vi "Analyze.vi"(8 "error in (no error)":errorcluster, 10 "Image in":T1, 11 "Analyze FF Spectrum in":refnum<class "Analyze FF Spectrum.lvclass">) -> (0 "error out":errorcluster, 1 "Result":refnum<class "Analyze Results Base.lvclass">, 2 "Image out":T1, 3 "Analyze FF Spectrum out":refnum<class "Analyze FF Spectrum.lvclass">)   [LabVIEW 2020, in "Analyze.lvlib" / "Analyze FF Spectrum.lvclass"]
uses:
  Analyze FF Spectrum.lvclass
  C:/POLARIS Programme/POLARIS-AS-3-Cams/Submodules/HIJ Vision/Analyze/Analyze Classes/Analyze BaseClass/Analyze BaseClass/Analyze BaseClass.lvclass
  <vilib>/vision/Image Controls.llb/IMAQ Image.ctl
  Results and Overlays/Results Base/Analyze Results Base.lvclass
  Results and Overlays/Results SRFF/Analyze Results FF-Spectrum.lvclass
  C:/POLARIS Programme/POLARIS-AS-3-Cams/Submodules/HIJ Vision/Analyze/Results and Overlays/Results Base/Analyze Results Base.lvclass
  Analyze Parameter/Analyze Parameter Spectral Calibration/Analyze Parameter Spectral Calibration.lvclass
  C:/POLARIS Programme/POLARIS-AS-3-Cams/Submodules/HIJ Vision/Analyze/Analyze Parameter/Analyze Parameter Base/Analyze Parameter Base.lvclass
  Results and Overlays/Results SRFF/Analyze Results FF-Spectrum.lvclass/Analyze Results FF-Spectrum.ctl
  Results and Overlays/Results SRFF/Write SRFF Spectrum.vi
  Analyze BaseClass/Analyze BaseClass/Analyze BaseClass.lvclass
  <vilib>/vision/NI_Vision_Development_Module.lvlib
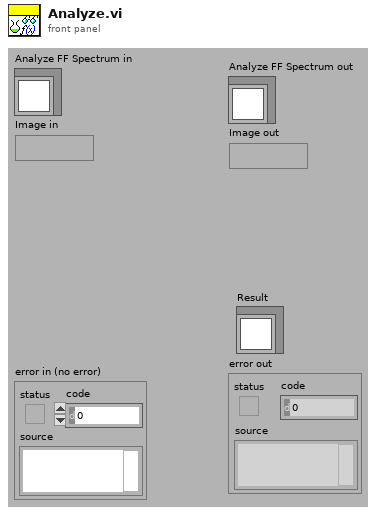
[diagram p1: front panel]
types:
  T1 = typedef "IMAQ Image.ctl" = refnum<image>
  T2 = typedef "Image Type" = u32
  T3 = typedef "ROI Descriptor" = cluster{"Global Rectangle":i32[], "Contours":cluster{"ID":enum32{"External", "Internal"}, "Type":u32, "Coordinates":i32[]}[]}
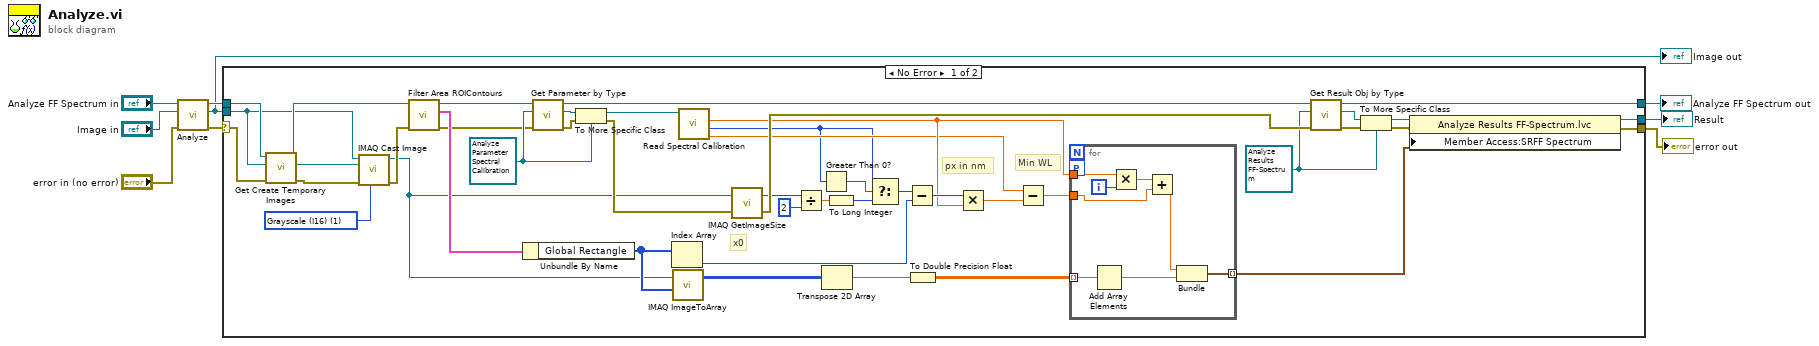
[diagram p0: block diagram]
diagram:
  n1 = call-parent "Analyze.vi"("error in (no error)"="error in (no error)", "Image in"="Image in", "Analyze BaseClass in"="Analyze FF Spectrum in") -> ("error out"=w1:errorcluster, "Image out"=w6:T1, "Analyze BaseClass out"=w7:refnum<class "Analyze FF Spectrum.lvclass">)  [unwired: 5 in, 1 out]
  "Image out" <- w6
  n2 = case shown="No Error" w1 {
    selector: w1 -> [w17 w64]
    tunnel: w7 -> [w18 w63]
    tunnel: w6 -> [w13 _]
    tunnel: [w34 _] -> w4
    tunnel: [w33 w64] -> w3
    tunnel: [w24 w63] -> w2
    frame No Error {
      w11 = T2 1 items=["Grayscale (U8)", "Grayscale (I16)", "Grayscale (SGL)", "Complex (CSG)", "RGB (U32)", "HSL (U32)", "RGB (U64)", "Grayscale (U16)"] ("Image Type")
      w29 = refnum<class "Analyze Parameter Spectral Calibration.lvclass"> refnum ("Spectral Calibration")
      w21 = refnum<class "Analyze Results FF-Spectrum.lvclass"> refnum ("Analyze Results FF-Spectrum.lvclass")
      # "px in nm"
      # "x0"
      # "Min WL"
      n3 = call-dynamic "Get Create Temporary Images.vi"("error in (no error)"=w17, "Image in"=w13, "Analyze BaseClass in"=w18) -> ("error out"=w15:errorcluster, "work image"=w12:T1, "Analyze BaseClass out"=w16:refnum<class "Analyze FF Spectrum.lvclass">)  [unwired: 4 in, 2 out]
      n4 = call "IMAQ Cast Image"("Image Type"=w11, "error in (no error)"=w15, "Image Dst"=w12, "Image Src"=w13) -> ("error out"=w14:errorcluster, "Image Dst Out"=w10:T1)  [unwired: 6 in]
      n5 = call-dynamic "Filter Area ROIContours.vi"("error in (no error)"=w14, "Analyze BaseClass in"=w16) -> ("error out"=w26:errorcluster, "ROI of Area type"=w53:T3, "Analyze BaseClass out"=w32:refnum<class "Analyze FF Spectrum.lvclass">)  [unwired: 7 in]
      n6 = Unbundle By Name(w53) -> ("Global Rectangle"=w47:i32[])
      n7 = call "Get Parameter by Type.vi"("error in (no error)"=w26, "Parameter Type"=w29, "Analyze BaseClass in"=w32) -> ("error out"=w27:errorcluster, "Parameter"=w28:refnum<class "Analyze Parameter Base.lvclass">, "Analyze BaseClass out"=w31:refnum<class "Analyze FF Spectrum.lvclass">)  [unwired: 5 in, 1 out]
      n8 = To More Specific Class(target class=w29, reference=w28, error in=w27) -> (specific class reference=w30:refnum<class "Analyze Parameter Spectral Calibration.lvclass">, error out=w25:errorcluster)
      n9 = Index Array(array=w47) -> (element=w46:i32)  [unwired: 1 in]
      n10 = call "IMAQ ImageToArray"("Optional Rectangle"=w47, "Image"=w10) -> ("Image Pixels (I16)"=w52:i16[][])  [unwired: 2 in, 4 out]
      n11 = call "Read Spectral Calibration.vi"("Analyze Parameter Spectral Calibration in"=w30) -> ("Central WL"=w40:dbl[unit], "Central Pixel"=w38:i32, "nm per px"=w41:dbl[unit])  [unwired: 7 in, 1 out]
      n12 = call "IMAQ GetImageSize"("Image"=w10, "error in (no error)"=w25) -> ("X Resolution"=w49:i32, "error out"=w54:errorcluster)  [unwired: 2 in, 1 out]
      n13 = Divide(x=w49, y=2) -> (x/y=w37:dbl)
      n14 = Greater Than 0?(x=w38) -> (x > 0?=w39:bool)
      n15 = Transpose 2D Array(2D array=w52) -> (transposed array=w50:i16[][])
      n16 = To Long Integer(number=w37) -> (32bit integer=w35:i32)
      n17 = Select(t=w38, s=w39, f=w35) -> (s? t:f=w36:i32)
      n18 = Subtract(x=w36, y=w46) -> (x-y=w45:i32)
      n19 = To Double Precision Float(number=w50) -> (double precision float=w51:dbl[][])
      n20 = Multiply(x=w45, y=w41) -> (x*y=w44:dbl[unit])
      n21 = Subtract(x=w40, y=w44) -> (x-y=w43:dbl[unit])
      n22 = for {
        tunnel: w51 -> [w62] mode=indexing
        tunnel: w43 -> [w58]
        tunnel: w41 -> [w60]
        tunnel: [w55] -> w42 mode=indexing
        workers-P: _ -> [_]
        i -> [w61]
        n23 = Add Array Elements(numeric array=w62) -> (sum=w56:dbl)
        n24 = Multiply(x=w60, y=w61) -> (x*y=w59:dbl[unit])
        n25 = Add(x=w59, y=w58) -> (x+y=w57:dbl[unit])
        n26 = Bundle(w57, w56) -> (w55:cluster{dbl[unit], dbl})  [unwired: 1 in]
      }
      n27 = call "Get Result Obj by Type.vi"("error in (no error)"=w54, "Parameter Type"=w21, "Analyze BaseClass in"=w31) -> ("error out"=w23:errorcluster, "Parameter"=w22:refnum<class "Analyze Results Base.lvclass">, "Analyze BaseClass out"=w24:refnum<class "Analyze FF Spectrum.lvclass">)  [unwired: 5 in, 1 out]
      n28 = To More Specific Class(target class=w21, reference=w22, error in=w23) -> (specific class reference=w20:refnum<class "Analyze Results FF-Spectrum.lvclass">, error out=w19:errorcluster)
      n29 = property class="Analyze Results FF-Spectrum.lvc"(reference=w20, error in=w19, "Member Access:SRFF Spectrum"=w42) -> (reference out=w34:refnum<class "Analyze Results FF-Spectrum.lvclass">, error out=w33:errorcluster)
    }
    frame Error {
    }
  }
  "error out" <- w3
  "Analyze FF Spectrum out" <- w2
  "Result" <- w4
